vi "ParBSend.vi"(0 "ref in":u64, 5 "R__ID":u32=1, 7 "Size":i32, 9 "Data":string, 11 "error in (no error)":errorcluster) -> (4 "ref out":u64, 6 "Result":i32, 15 "error out":errorcluster)   [LabVIEW 2018, in "Snap7.lvlib"]
uses:
  Snap7.lvlib
  windows/lv_snap7.dll
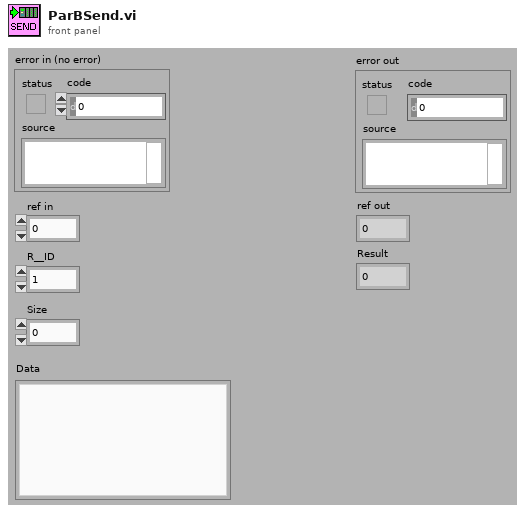
[diagram p1: front panel]
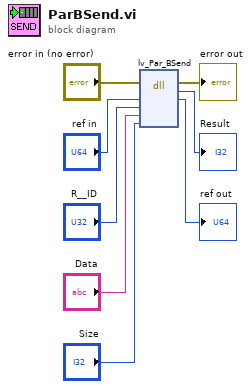
[diagram p0: block diagram]
diagram:
  n1 = dll-call lib="PTH2iabs D项目Feng恒隆项目Labview性能试验台SourcesSnap7libwindowslv_snap7.dll" fn="lv_Par_BSend"(error in="error in (no error)", "Partner"="ref in", "R_ID"="R__ID", "pUsrData"="Data", "Size"="Size") -> (error out=→"error out":errorcluster, "return type"=→"Result":i32, "Partner"=→"ref out":u64)  [unwired: 5 in, 1 out]
